vi "Relay Test_TS_v2.vi"(8 "error in (no error)":errorcluster, 11 "Control Board VISA":refnum<visa-resource-name>="ControlBoard") -> (0 "error out":errorcluster, 2 "Message OUT":string, 3 "Result (bool)":bool)   [LabVIEW 2022 SP3]
uses:
  <vilib>/DAQmx/read.llb/DAQmx Read (Digital 1D Bool NChan 1Samp 1Line).vi
  <vilib>/DAQmx/miscellaneous.llb/DAQmx Fill In Error Info.vi
panel:
  in  "Message IN":string
  out "Result (color)":u32(colorbox)
  out "cDAQ DI Reading":bool[](array[boolean])
  out "LC DO Cmd":bool[](array[boolean])
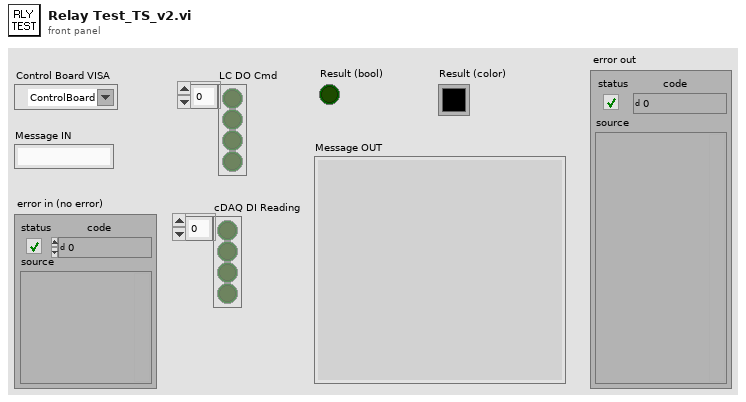
[diagram p1: front panel]
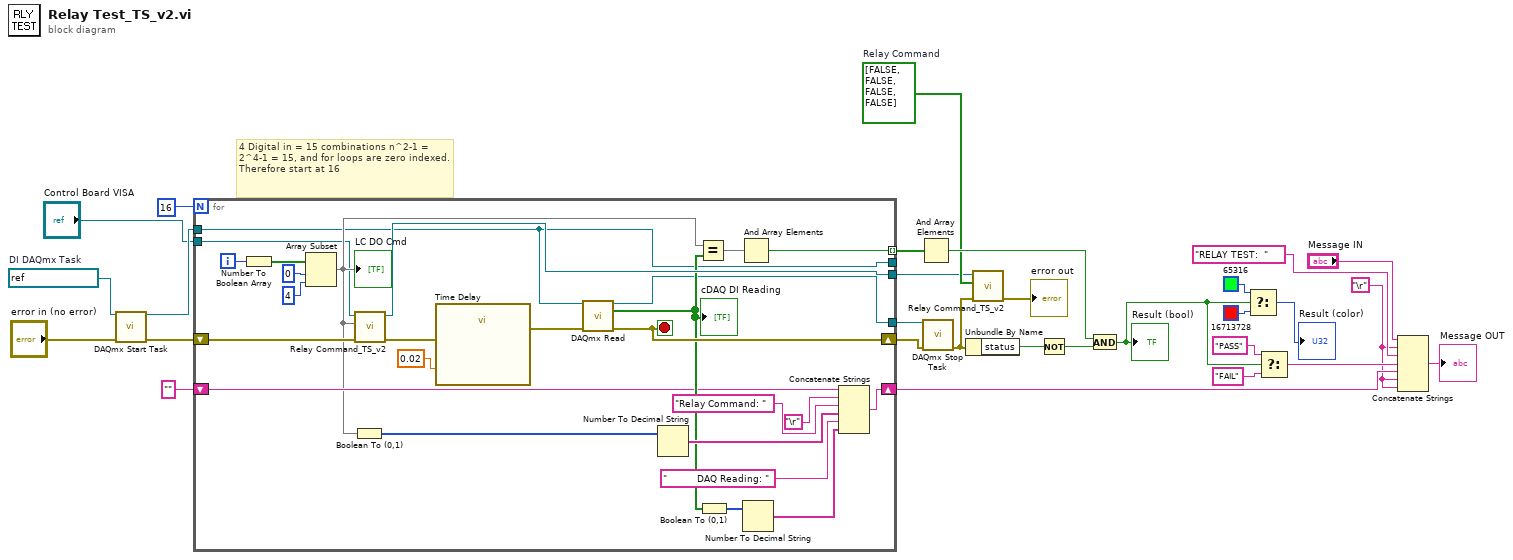
[diagram p0: block diagram]
diagram:
  w9 = refnum<k21> "BTS_RelayIn"  # DI DAQmx Task
  w10 = bool[] [FALSE, FALSE, FALSE, FALSE]  # Relay Command
  w13 = "\r"
  # "4 Digital in = 15 combinations n^2-1 = 2^4-1 = 15, and for loops are zero indexed.  Therefore start at 16"
  n1 = call <vilib>:"DAQmx Start Task.vi"("task/channels in"=w9, "error in"="error in (no error)") -> ("task out"=w8:refnum<k21>, "error out"=w6:errorcluster)  [unwired: 12 in]
  n2 = for {
    N: 16 -> [_]
    shift-right: [w49] -> w5
    shift-left: w6 -> [w53]
    tunnel: [w51] -> w1
    tunnel: [w55] -> w29 mode=indexing
    shift-right: [w37] -> w17
    shift-left: "" -> [w36]
    tunnel: [w33] -> _
    tunnel: w8 -> [w33]
    tunnel: [w32] -> w3
    tunnel: "Control Board VISA" -> [w31]
    i -> [w35]
    stop <- w49 stop-if-true
    n3 = Number To Boolean Array(number=w35) -> (Boolean array=w39:bool[])
    n4 = Array Subset(array=w39, index=0, length=4) -> (w34:bool[])
    "LC DO Cmd" <- w34
    n5 = Boolean To (0,1)(Boolean=w34) -> (0, 1=w43:i16[])
    n6 = call "Relay Command_TS_v2.vi"("error in (no error)"=w53, "Relay Command"=w34, "Control Board VISA"=w31) -> ("error out"=w52:errorcluster, "VISA Refnum out"=w51:refnum<visa-resource-name>)  [unwired: 7 in]
    n7 = call "Time Delay"("error in (no error)"=w52, "Delay Time (s)"=0.02) -> ("error out"=w50:errorcluster)  [unwired: 9 in]
    n8 = call-poly <vilib>:"DAQmx Read.vi"("task/channels in"=w33, "error in"=w50) -> ("task out"=w32:refnum<k21>, "data"=w38:bool[], "error out"=w49:errorcluster)  [unwired: 11 in]
    "cDAQ DI Reading" <- w38
    n9 = Number To Decimal String(number=w43) -> (decimal integer string=w46:string[])  [unwired: 1 in]
    n10 = Equal?(x=w34, y=w38) -> (x = y?=w54:bool[])
    n11 = Boolean To (0,1)(Boolean=w38) -> (0, 1=w42:i16[])
    n12 = And Array Elements(Boolean array=w54) -> (logical AND=w55:bool)
    n13 = Number To Decimal String(number=w42) -> (decimal integer string=w48:string[])  [unwired: 1 in]
    n14 = Concatenate Strings(w36, "\r", "Relay Command: ", w46, "          DAQ Reading: ", w48) -> (w37:string)
  }
  n15 = And Array Elements(Boolean array=w29) -> (logical AND=w19:bool)
  n16 = call <vilib>:"DAQmx Stop Task.vi"("task/channels in"=w3, "error in"=w5) -> ("error out"=w4:errorcluster)  [unwired: 12 in, 1 out]
  n17 = Unbundle By Name(w4) -> ("status"=w22:bool)
  n18 = call "Relay Command_TS_v2.vi"("error in (no error)"=w4, "Relay Command"=w10, "Control Board VISA"=w1) -> ("error out"=→"error out":errorcluster)  [unwired: 7 in, 1 out]
  n19 = Not(x=w22) -> (.not. x?=w21:bool)
  n20 = And(x=w19, y=w21) -> (x .and. y?=w20:bool)
  "Result (bool)" <- w20
  n21 = Select(t=u32 65316 ("Result (color)"), s=w20, f=u32 16713728 ("Result (color)")) -> (s? t:f=→"Result (color)":u32)
  n22 = Select(t="PASS", s=w20, f="FAIL") -> (s? t:f=w16:string)
  n23 = Concatenate Strings("Message IN", w13, "RELAY TEST:  ", w16, w17, w13, w13) -> (→"Message OUT":string)
